vi "flowSensor.vi"() -> ()   [LabVIEW 2023]
uses:
  <vilib>/DAQmx/read.llb/DAQmx Read (Analog DBL 1Chan 1Samp).vi
  <vilib>/DAQmx/create/channels.llb/DAQmx Create Channel (AI-Voltage-Basic).vi
  <vilib>/DAQmx/configure/timing.llb/DAQmx Timing (Sample Clock).vi
  <vilib>/DAQmx/miscellaneous.llb/DAQmx Fill In Error Info.vi
  <vilib>/ptbypt/NI_PtbyPt.lvlib
panel:
  in  "Measurement Interval (sec)":dbl=5.0 caption="Time Target (s)"
  out "LPM":dbl
  out "Elapsed Time (s)":dbl
  out "pulses":i32
  out "Waveform Chart":dbl(graph)
  in  "?":bool
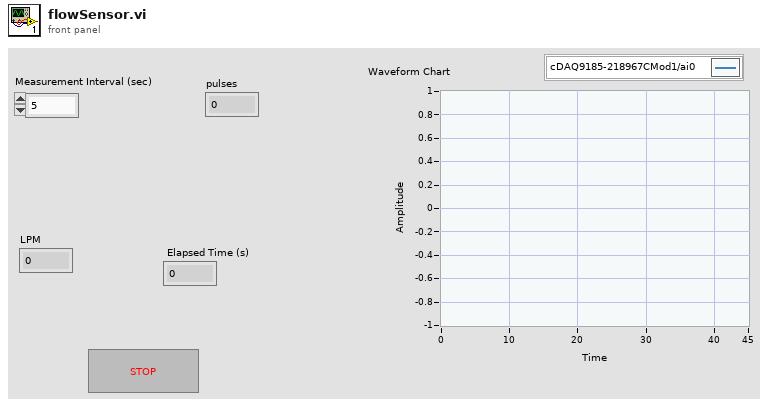
[diagram p1: front panel]
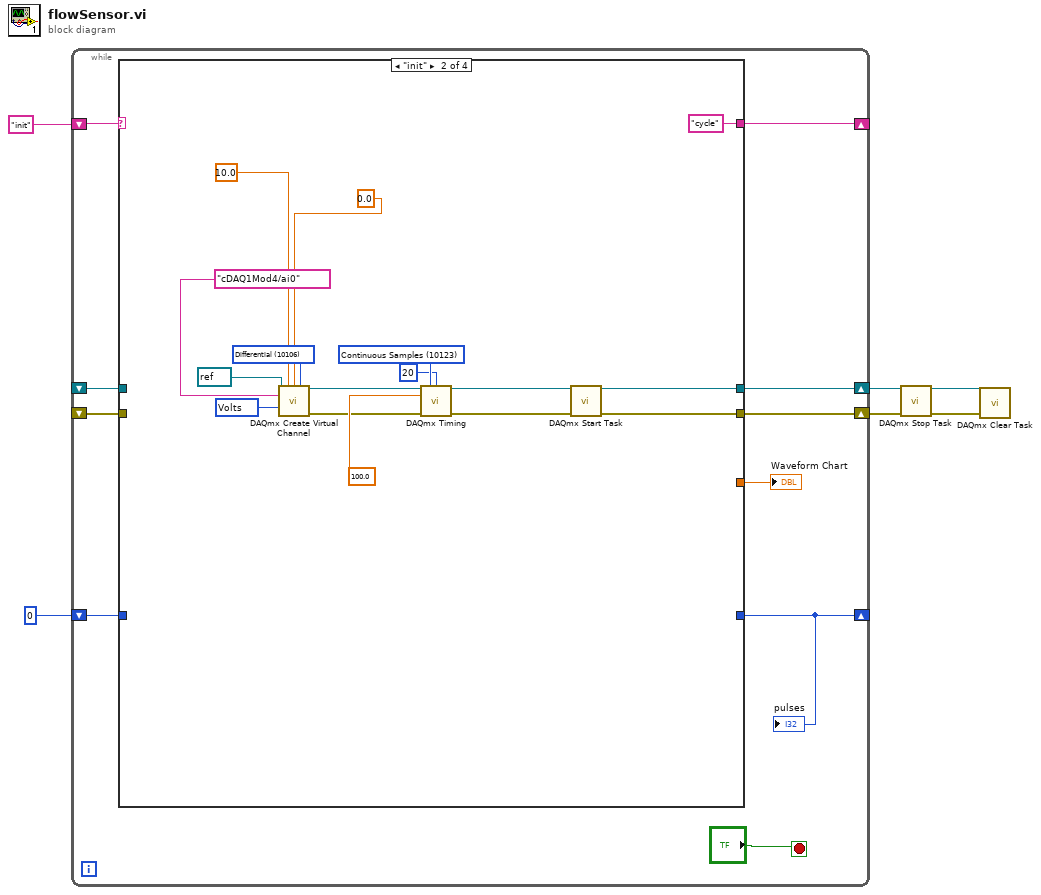
[diagram p0: block diagram]
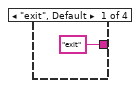
[diagram p2: hidden frame]
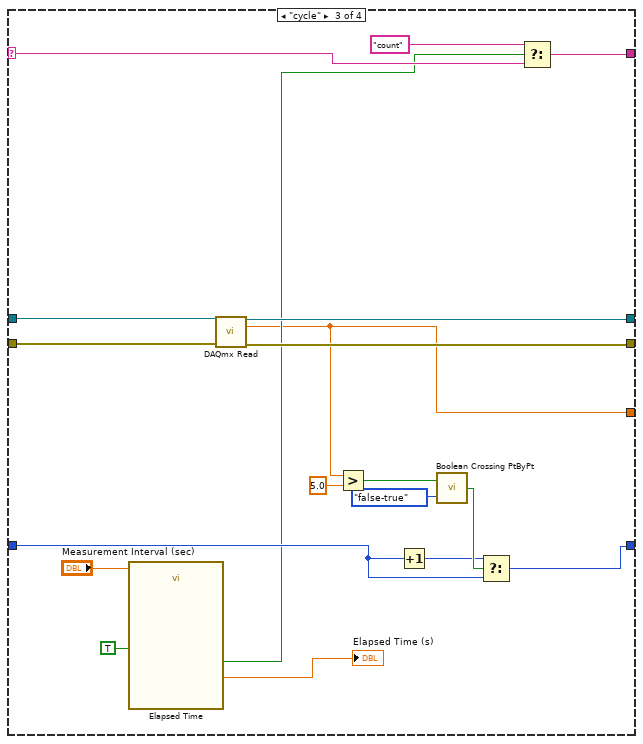
[diagram p3: hidden frame]
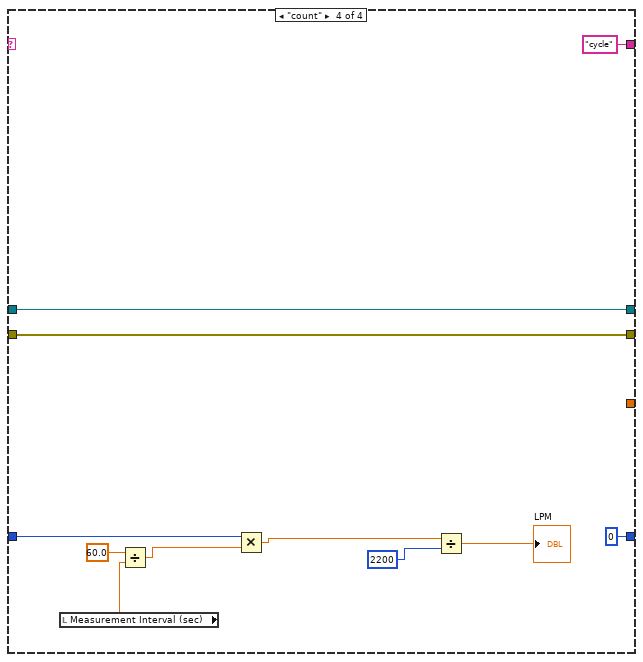
[diagram p4: hidden frame]
diagram:
  n1 = while {
    shift-right: [w15] -> _
    shift-left: "init" -> [w16]
    shift-right: [w14] -> w6
    shift-left: _ -> [w12]
    shift-right: [w13] -> w5
    shift-left: _ -> [w11]
    shift-right: [w9] -> _
    shift-left: 0 -> [w10]
    stop <- "?" stop-if-true
    n2 = case shown="\"init\"" w16 {
      selector: w16 -> [_ _ w40 _]
      tunnel: ["exit" "cycle" w41 "cycle"] -> w15
      tunnel: [_ w19 w51 w61] -> w14
      tunnel: [_ w18 w52 w60] -> w13
      tunnel: w12 -> [_ _ w50 w61]
      tunnel: w11 -> [_ _ w49 w60]
      tunnel: [_ _ w42 0] -> w9
      tunnel: w10 -> [_ _ w43 w58]
      tunnel: [_ _ w34 _] -> w7
      frame "exit", Default {
      }
      frame "init" {
        w28 = 10123 items=["Finite Samples"=10178, "Continuous Samples"=10123, "Hardware Timed Single Point"=12522] ("sample mode")
        w29 = 10106 items=["Default"=-1, "RSE"=10083, "NRSE"=10078, "Differential"=10106, "Pseudodifferential"=12529] ("input terminal configuration")
        w30 = 10348 items=["Volts"=10348, "From Custom Scale"=10065] ("units")
        n3 = call-poly <vilib>:"DAQmx Create Virtual Channel.vi"("task in"=refnum<k21> refnum, "maximum value"=10.0 ("minimum value"), "minimum value"=0.0, "input terminal configuration"=w29, "physical channels"=tag "cDAQ1Mod4/ai0", "units"=w30) -> ("task out"=w24:refnum<k21>, "error out"=w23:errorcluster)  [unwired: 8 in]
        n4 = call-poly <vilib>:"DAQmx Timing.vi"("task/channels in"=w24, "sample mode"=w28, "samples per channel"=20, "rate"=100.0, "error in"=w23) -> ("task out"=w21:refnum<k21>, "error out"=w20:errorcluster)  [unwired: 9 in]
        n5 = call <vilib>:"DAQmx Start Task.vi"("task/channels in"=w21, "error in"=w20) -> ("task out"=w19:refnum<k21>, "error out"=w18:errorcluster)  [unwired: 12 in]
      }
      frame "cycle" {
        n6 = call "Elapsed Time"("Time Target (s)"="Measurement Interval (sec)", "Auto Reset"=TRUE) -> ("Elapsed Time (s)"=→"Elapsed Time (s)":dbl, "Time has Elapsed"=w35:bool)  [unwired: 10 in, 6 out]
        n7 = call-poly <vilib>:"DAQmx Read.vi"("task/channels in"=w50, "error in"=w49) -> ("task out"=w51:refnum<k21>, "data"=w34:dbl, "error out"=w52:errorcluster)  [unwired: 11 in]
        n8 = Greater?(x=w34, y=5.0) -> (0:w47:bool)
        n9 = Increment(x=w43) -> (x+1=w44:i32)
        n10 = call <vilib>:"Boolean Crossing PtByPt.vi"("direction"=enum16{"either", "false-true", "true-false"}."false-true", "input"=w47) -> ("crossing"=w45:bool)  [unwired: 1 in]
        n11 = Select(t=w44, s=w45, f=w43) -> (s? t:f=w42:i32)
        n12 = Select(t="count", s=w35, f=w40) -> (s? t:f=w41:string)
      }
      frame "count" {
        n13 = local read "Measurement Interval (sec)"() -> (w54:dbl)
        n14 = Divide(x=60.0, y=w54) -> (x/y=w56:dbl)
        n15 = Multiply(x=w58, y=w56) -> (x*y=w57:dbl)
        n16 = Divide(x=w57, y=2200) -> (x/y=→"LPM":dbl)
      }
    }
    "pulses" <- w9
    "Waveform Chart" <- w7
  }
  n17 = call <vilib>:"DAQmx Stop Task.vi"("task/channels in"=w6, "error in"=w5) -> ("task out"=w4:refnum<k21>, "error out"=w3:errorcluster)  [unwired: 12 in]
  n18 = call <vilib>:"DAQmx Clear Task.vi"("task in"=w4, "error in"=w3) -> ()  [unwired: 13 in, 1 out]
